vi "remove fom info from sysdef tree.vi"(8 "error in":errorcluster, 11 "Item Ref in":T1 format="%.0x") -> (0 "error out":errorcluster, 3 "Item Ref out":T1 format="%.0x")   [LabVIEW 2019, in "HLA Custom Device System Explorer.lvlib"]
uses:
  HLA Custom Device System Explorer.lvlib
  <vilib>/NI VeriStand/Custom Device API/Custom Device Item Ref.ctl
  <vilib>/NI VeriStand/Custom Device API/Custom Device API.lvlib
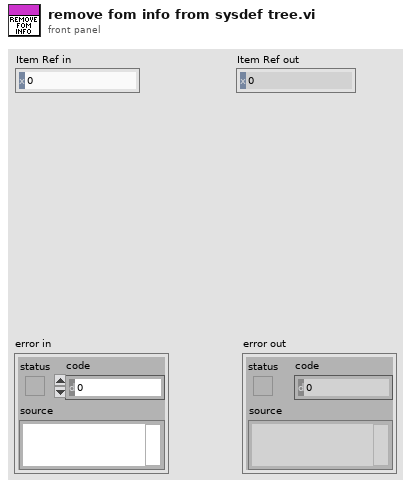
[diagram p1: front panel]
types:
  T1 = typedef "Custom Device API.lvlib/Custom Device Item Ref.ctl" = u64
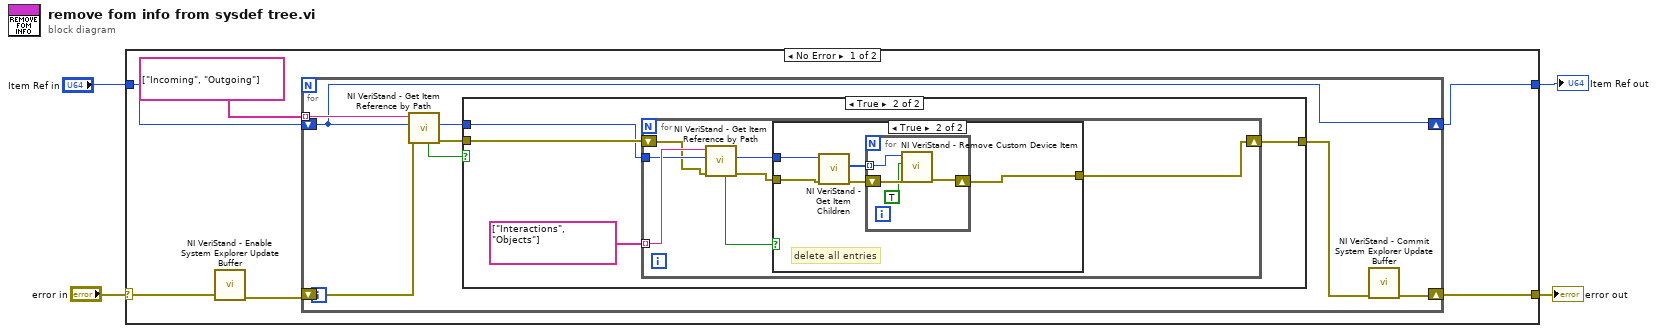
[diagram p0: block diagram]
diagram:
  n1 = case shown="No Error" "error in" {
    selector: "error in" -> [w6 w41]
    tunnel: [w8 w41] -> w3
    tunnel: [w7 w42] -> w2
    tunnel: "Item Ref in" -> [w10 w42]
    frame No Error {
      n2 = call <vilib>:"NI VeriStand - Enable System Explorer Update Buffer.vi"("error in (no error)"=w6) -> ("error out"=w5:errorcluster)  [unwired: 10 in]
      n3 = for {
        tunnel: string[] ["Incoming", "Outgoing"] ("Item Path in") -> [w17] mode=indexing
        shift-right: [w16] -> w7
        shift-left: w10 -> [w16]
        shift-right: [w11] -> w8
        shift-left: w5 -> [w18]
        n4 = call <vilib>:"NI VeriStand - Get Item Reference by Path.vi"("error in (no error)"=w18, "Root Ref"=w16, "Item Path in"=w17) -> ("error out"=w13:errorcluster, "Item Ref"=w14:T1, "Found"=w15:bool)  [unwired: 5 in, 1 out]
        n5 = case shown="True" w15 {
          tunnel: w14 -> [_ w21]
          tunnel: w13 -> [w19 w23]
          tunnel: [w19 w20] -> w12
          frame False {
          }
          frame True {
            n6 = for {
              shift-right: [w24] -> w20
              shift-left: w23 -> [w25]
              tunnel: string[] ["Interactions", "Objects"] ("Item Path in") -> [w30] mode=indexing
              tunnel: w21 -> [w29]
              n7 = call <vilib>:"NI VeriStand - Get Item Reference by Path.vi"("error in (no error)"=w25, "Root Ref"=w29, "Item Path in"=w30) -> ("error out"=w26:errorcluster, "Item Ref"=w27:T1, "Found"=w28:bool)  [unwired: 5 in, 1 out]
              n8 = case shown="True" w28 {
                tunnel: w27 -> [_ w36]
                tunnel: w26 -> [w31 w35]
                tunnel: [w31 w32] -> w24
                frame False {
                }
                frame True {
                  # "delete all entries"
                  n9 = call <vilib>:"NI VeriStand - Get Item Children.vi"("error in (no error)"=w35, "Item Ref in"=w36) -> ("error out"=w34:errorcluster, "Child Refs"=w33:T1[])  [unwired: 6 in, 2 out]
                  n10 = for {
                    shift-right: [w38] -> w32
                    shift-left: w34 -> [w40]
                    tunnel: w33 -> [w39] mode=indexing
                    n11 = call <vilib>:"NI VeriStand - Remove Custom Device Item.vi"("error in (no error)"=w40, "Force Delete (F)"=TRUE, "Item Ref in"=w39) -> ("error out"=w38:errorcluster)  [unwired: 7 in, 1 out]
                  }
                }
              }
            }
          }
        }
        n12 = call <vilib>:"NI VeriStand - Commit System Explorer Update Buffer.vi"("error in (no error)"=w12) -> ("error out"=w11:errorcluster)  [unwired: 10 in]
      }
    }
    frame Error {
    }
  }
  "error out" <- w3
  "Item Ref out" <- w2
